vi "CopyMemory.vi"(4 "error in (no error)":errorcluster, 5 "length (0)":u32, 6 "hMemDestination (NULL)":i32, 7 "hMemSource (NULL)":i32) -> (0 "error out":errorcluster)   [LabVIEW 2011]
uses:
  KERNEL32.DLL
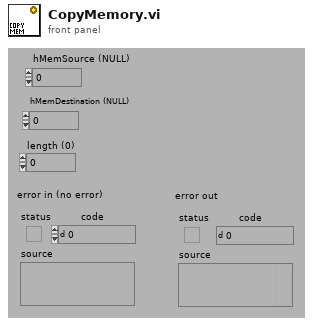
[diagram p1: front panel]
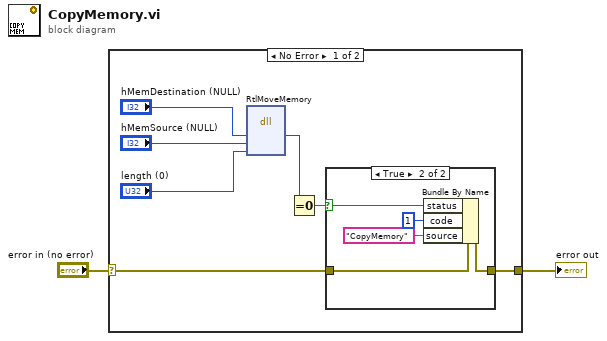
[diagram p0: block diagram]
diagram:
  n1 = case shown="No Error" "error in (no error)" {
    selector: "error in (no error)" -> [w8 w16]
    tunnel: [w7 w16] -> w1
    frame No Error {
      n2 = dll-call lib="KERNEL32.DLL" fn="RtlMoveMemory" label="void CopyMemory(\n     unsigned long pDestination, \n     unsigned long pSource, unsigned long length);"("hMemDestination (NULL)"="hMemDestination (NULL)", "hMemSource (NULL)"="hMemSource (NULL)", "length"="length (0)") -> ("hMemDestination (NULL)"=w3:i32)  [unwired: 5 in, 3 out]
      n3 = Equal To 0?(x=w3) -> (x = 0?=w9:bool)
      n4 = case shown="True" w9 {
        selector: w9 -> [_ w14]
        tunnel: w8 -> [w10 w15]
        tunnel: [w10 w13] -> w7
        frame False {
        }
        frame True {
          n5 = Bundle By Name(cluster=w15, "status"=w14, "code"=1, "source"="CopyMemory") -> (w13:errorcluster)
        }
      }
    }
    frame Error {
    }
  }
  "error out" <- w1
